vi "_RT_Check_Startup_Time.vi"() -> ()   [LabVIEW 2018]
panel:
  out "error out":errorcluster={"status"=TRUE, "code"=5004, "source"="Ping TimeOut"}
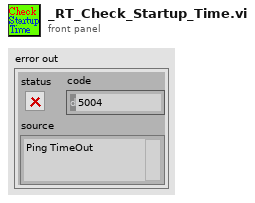
[diagram p1: front panel]
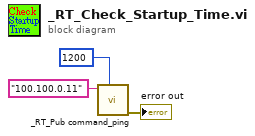
[diagram p0: block diagram]
diagram:
  n1 = call "_RT_Pub command_ping.vi"("Loop Times"=1200, "PCIP String"="100.100.0.11") -> ("error out"=→"error out":errorcluster)  [unwired: 9 in]
